vi "Get Node Ref.vi"(8 "error in (no error)":errorcluster, 9 "y":i32, 10 "x":i32, 11 "OccupancyGridWorldMap in":refnum<class "NI_Robotics_OccupancyGridWorldMap.lvclass">) -> (0 "error out":errorcluster, 1 "Found":bool, 2 "element":refnum<data-value>, 3 "OccupancyGridWorldMap out":refnum<class "NI_Robotics_OccupancyGridWorldMap.lvclass">)   [LabVIEW 2017, in "NI_Robotics_OccupancyGridWorldMap.lvclass"]
uses:
  <vilib>/robotics/Navigation/shared/WorldMap/OccupancyGridWorldMap/NI_Robotics_OccupancyGridWorldMap.lvclass
  <vilib>/robotics/Navigation/shared/MapNode/OccupancyGridNode/NI_Robotics_OccupancyGridMapNode.lvclass
  <vilib>/robotics/Navigation/shared/WorldMap/OccupancyGridWorldMap/NI_Robotics_OccupancyGridWorldMap.lvclass/NI_Robotics_OccupancyGridWorldMap.ctl
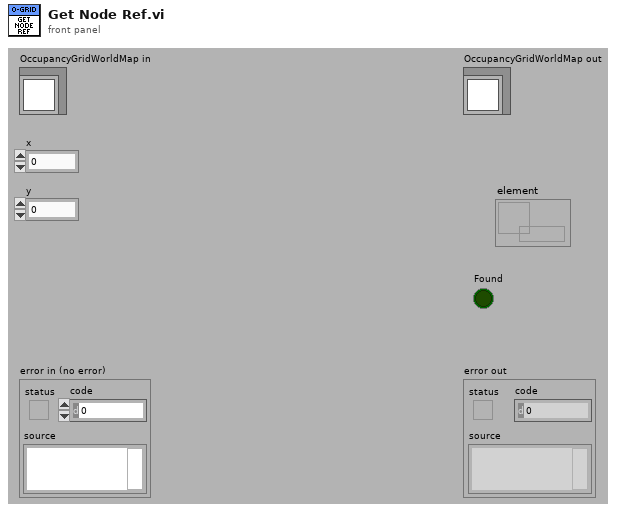
[diagram p1: front panel]
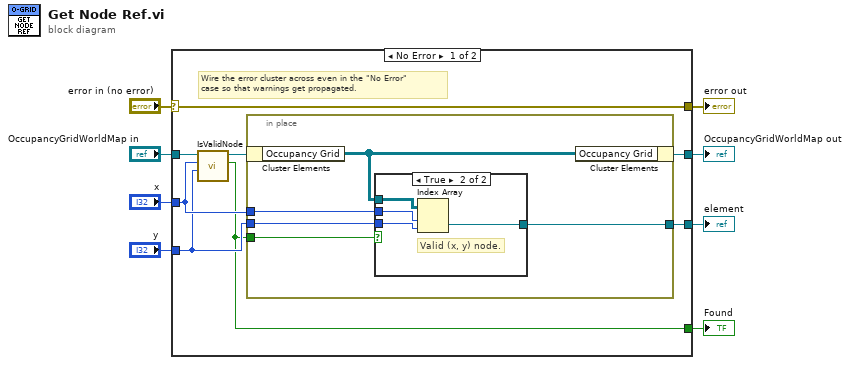
[diagram p0: block diagram]
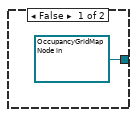
[diagram p2: hidden frame]
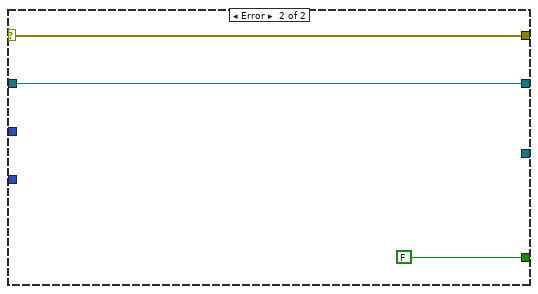
[diagram p3: hidden frame]
diagram:
  n1 = case shown="No Error" "error in (no error)" {
    selector: "error in (no error)" -> [w16 w29]
    tunnel: [w16 w29] -> w7
    tunnel: [w14 w28] -> w5
    tunnel: "OccupancyGridWorldMap in" -> [w13 w28]
    tunnel: "x" -> [w11 _]
    tunnel: "y" -> [w10 _]
    tunnel: [w15 _] -> w2
    tunnel: [w9 FALSE] -> w1
    frame No Error {
      # "Wire the error cluster across even in the \"No Error\"\ncase so that warnings get propagated."
      n2 = call <vilib>:"IsValidNode.vi"("y"=w10, "x"=w11, "OccupancyGridWorldMap in"=w13) -> ("Valid"=w9:bool, "OccupancyGridWorldMap out"=w12:refnum<class "NI_Robotics_OccupancyGridWorldMap.lvclass">)  [unwired: 7 in]
      n3 = in-place {
        in-place-border: w11 -> [w19]
        in-place-border: w10 -> [w18]
        in-place-border: [w21] -> w15
        in-place-border: w9 -> [w17]
        n4 = in-place-cluster #1(w12) -> ("Occupancy Grid"=w20:refnum<data-value>[][])
        n5 = case shown="True" w17 {
          tunnel: [refnum<data-value> refnum ("data value reference") w26] -> w21
          tunnel: w20 -> [_ w25]
          tunnel: w19 -> [_ w24]
          tunnel: w18 -> [_ w23]
          frame False {
          }
          frame True {
            # "Valid (x, y) node."
            n6 = Index Array(array=w25, index (row)=w24, index (col)=w23) -> (element=w26:refnum<data-value>)
          }
        }
        n7 = in-place-cluster #1("Occupancy Grid"=w20) -> (w14:refnum<class "NI_Robotics_OccupancyGridWorldMap.lvclass">)
      }
    }
    frame Error {
    }
  }
  "error out" <- w7
  "OccupancyGridWorldMap out" <- w5
  "element" <- w2
  "Found" <- w1
